vi "Initialize.vi"(8 "error in (no error)":errorcluster, 11 "VICI Electronic Actuator In":T1) -> (0 "error out":errorcluster, 1 "Initialized":bool, 2 "No Valve Connected":bool, 3 "VICI Electronic Actuator Out":T1)   [LabVIEW 2018, in "VICI Electronic Actuator.lvlib"]
uses:
  D-O Module Folder/DIO Valve/VICI Electronic Actuator.lvlib
  VICI Electronic Actuator Settings.ctl
  <vilib>/Instr/_visa.llb/VISA Configure Serial Port (Instr).vi
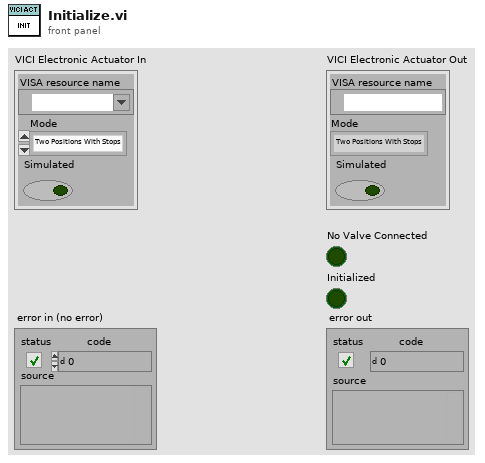
[diagram p1: front panel]
types:
  T1 = typedef "VICI Electronic Actuator.lvlib/VICI Electronic Actuator Settings.ctl" = cluster{"VISA resource name":refnum<visa-resource-name>, "Mode":enum16{"Two Positions With Stops", "Two Positions Without Stops", "Mutiposition"}, "Simulated":bool}
  T2 = enum16{"Two Positions With Stops", "Two Positions Without Stops", "Mutiposition"}
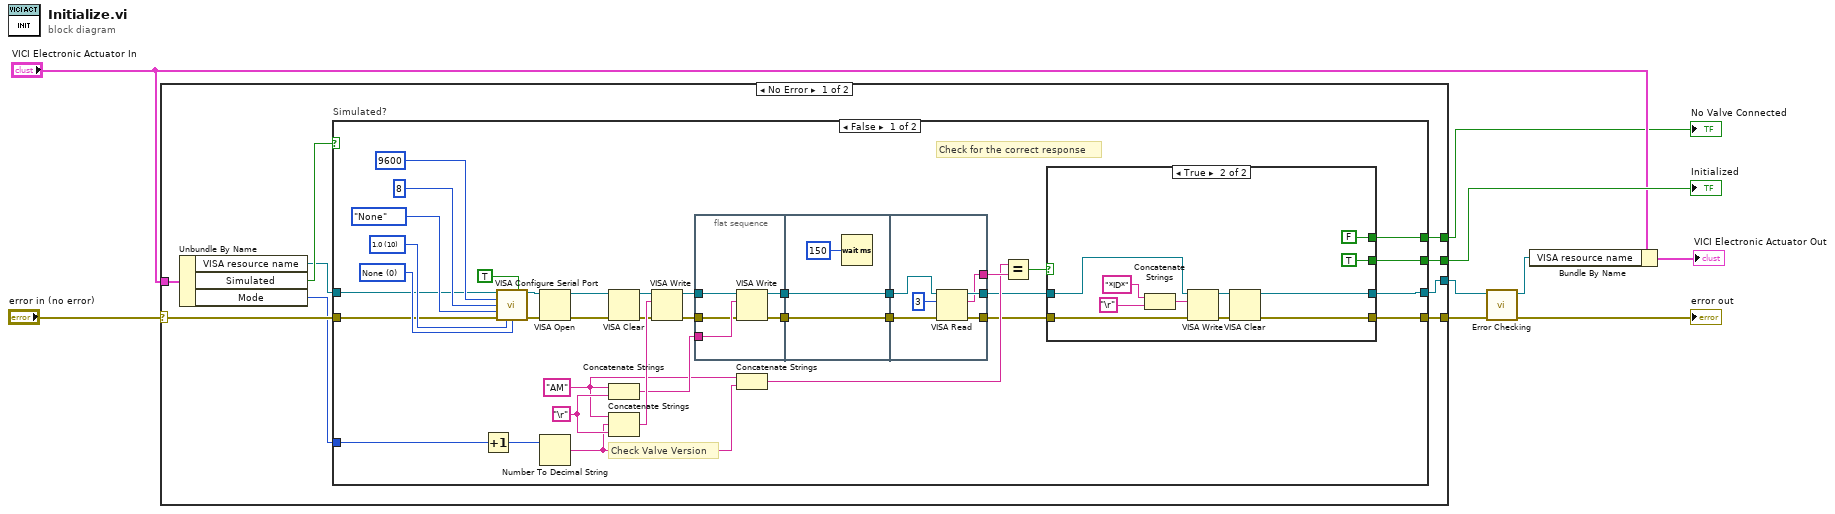
[diagram p0: block diagram]
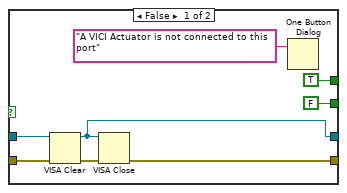
[diagram p2: hidden frame]
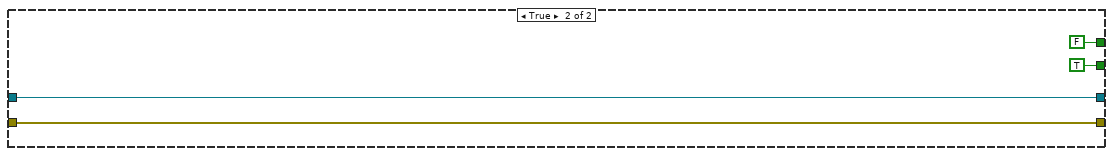
[diagram p3: hidden frame]
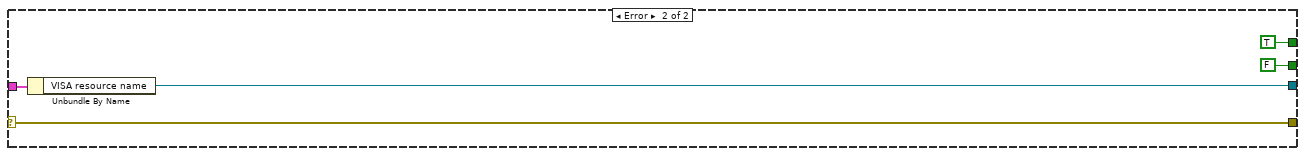
[diagram p4: hidden frame]
diagram:
  n1 = case shown="No Error" "error in (no error)" {
    selector: "error in (no error)" -> [w18 w96]
    tunnel: "VICI Electronic Actuator In" -> [w15 w95]
    tunnel: [w16 w96] -> w7
    tunnel: [w13 w94] -> w8
    tunnel: [w11 FALSE] -> w4
    tunnel: [w10 TRUE] -> w1
    frame No Error {
      n2 = Unbundle By Name(w15) -> ("VISA resource name"=w14:refnum<visa-resource-name>, "Simulated"=w17:bool, "Mode"=w12:T2)
      n3 = case "Simulated?" shown="False" w17 {
        tunnel: w18 -> [w48 w91]
        tunnel: [w20 w91] -> w16
        tunnel: [w21 w90] -> w13
        tunnel: w14 -> [w46 w90]
        tunnel: w12 -> [w37 _]
        tunnel: [w38 TRUE] -> w11
        tunnel: [w19 FALSE] -> w10
        frame False {
          w26 = "AM" ("string")
          w29 = "\r"
          w50 = u16 0 items=["None", "XON/XOFF", "RTS/CTS", "XON/XOFF & RTS/CTS", "DTR/DSR", "XON/XOFF & DTR/DSR"] ("flow control (0:none)")
          w51 = u16 10 items=["1.0"=10, "1.5"=15, "2.0"=20] ("stop bits (10: 1 bit)")
          # "Check for the correct response"
          # "Check Valve Version"
          n4 = Increment(x=w37) -> (x+1=w36:T2)
          n5 = call-poly "VISA Configure Serial Port"("VISA resource name"=w46, "Enable Termination\nChar (T)"=TRUE ("Enable Termination\nChar (T)"), "baud rate (9600)"=u32 9600, "data bits (8)"=u16 8, "parity (0:none)"=enum16{"None", "Odd", "Even", "Mark", "Space"}."None", "error in (no error)"=w48, "stop bits (10: 1 bit)"=w51, "flow control (0:none)"=w50) -> ("VISA resource name out"=w47:refnum<visa-resource-name>, "error out"=w49:errorcluster)  [unwired: 6 in]
          n6 = VISA Open(error in (no error)=w49, VISA resource name=w47) -> (VISA resource name=w43:refnum<visa-resource-name>, error out=w40:errorcluster)  [unwired: 3 in]
          n7 = Number To Decimal String(number=w36) -> (decimal integer string=w27:string)  [unwired: 1 in]
          n8 = VISA Clear(VISA resource name=w43, error in (no error)=w40) -> (VISA resource name out=w42:refnum<visa-resource-name>, error out=w41:errorcluster)
          n9 = Concatenate Strings(w26, w29) -> (w28:string)
          n10 = Concatenate Strings(w26, w27, w29) -> (w44:string)
          n11 = VISA Write(VISA resource name=w42, write buffer=w44, error in (no error)=w41) -> (VISA resource name out=w31:refnum<visa-resource-name>, error out=w30:errorcluster)  [unwired: 1 out]
          n12 = flat-sequence {
            tunnel: w28 -> [w59]
            tunnel: [w58] -> w35
            tunnel: [w57] -> w34
            tunnel: w31 -> [w56]
            tunnel: w30 -> [w55]
            tunnel: [w61] -> w33
            tunnel: w35 -> [w61]
            tunnel: w34 -> [w60]
            tunnel: [w60] -> w32
            tunnel: [w68] -> w22
            tunnel: [w67] -> w23
            tunnel: w33 -> [w65]
            tunnel: w32 -> [w64]
            tunnel: [w63] -> w25
            frame #0 {
              n13 = VISA Write(VISA resource name=w56, write buffer=w59, error in (no error)=w55) -> (VISA resource name out=w58:refnum<visa-resource-name>, error out=w57:errorcluster)  [unwired: 1 out]
            }
            frame #1 {
              n14 = Wait (ms)(milliseconds to wait=u32 150) -> ()  [unwired: 1 out]
            }
            frame #2 {
              n15 = VISA Read(VISA resource name=w65, byte count=u32 3, error in (no error)=w64) -> (VISA resource name out=w67:refnum<visa-resource-name>, read buffer=w63:string, error out=w68:errorcluster)  [unwired: 1 out]
            }
          }
          n16 = Concatenate Strings(w26, w27) -> (w24:string)
          n17 = Equal?(x=w24, y=w25) -> (x = y?=w45:bool)
          n18 = case shown="True" w45 {
            tunnel: w23 -> [w70 w85]
            tunnel: w22 -> [w72 w84]
            tunnel: [TRUE FALSE] -> w19
            tunnel: [w74 w80] -> w20
            tunnel: [FALSE TRUE] -> w38
            tunnel: [w69 w81] -> w21
            frame False {
              n19 = VISA Clear(VISA resource name=w70, error in (no error)=w72) -> (VISA resource name out=w69:refnum<visa-resource-name>, error out=w71:errorcluster)
              n20 = VISA Close(VISA resource name=w69, error in (no error)=w71) -> (error out=w74:errorcluster)
              n21 = One Button Dialog(message="A VICI Actuator is not connected to this port") -> ()  [unwired: 1 in, 1 out]
            }
            frame True {
              n22 = Concatenate Strings("*ID*" ("string"), "\r") -> (w77:string)
              n23 = VISA Write(VISA resource name=w85, write buffer=w77, error in (no error)=w84) -> (VISA resource name out=w82:refnum<visa-resource-name>, error out=w83:errorcluster)  [unwired: 1 out]
              n24 = VISA Clear(VISA resource name=w82, error in (no error)=w83) -> (VISA resource name out=w81:refnum<visa-resource-name>, error out=w80:errorcluster)
            }
          }
        }
        frame True {
        }
      }
    }
    frame Error {
      n25 = Unbundle By Name(w95) -> ("VISA resource name"=w94:refnum<visa-resource-name>)
    }
  }
  "Initialized" <- w4
  "No Valve Connected" <- w1
  n26 = call "Error Checking.vi"("error in (no error)"=w7, "VISA resource name"=w8) -> ("error out"=→"error out":errorcluster, "VISA resource name"=w5:refnum<visa-resource-name>)  [unwired: 7 in, 1 out]
  n27 = Bundle By Name(cluster="VICI Electronic Actuator In", "VISA resource name"=w5) -> (→"VICI Electronic Actuator Out":T1)
